vi "Compress.vi"(4 "No of threads":i32, 6 "Compression Level":i32=3, 8 "error in (no error)":errorcluster, 11 "lvzstd in":refnum<class "lvzstd.lvclass">) -> (0 "error out":errorcluster, 3 "lvzstd out":refnum<class "lvzstd.lvclass">)   [LabVIEW 2020, in "lvzstd.lvlib" / "lvzstd.lvclass"]
uses:
  lvzstd.lvclass
  lvzstd.lvclass/lvzstd.ctl
  <vilib>/Utility/error.llb/Error Cluster From Error Code.vi
panel:
  in  "data in":variant
  out "compressed data":string
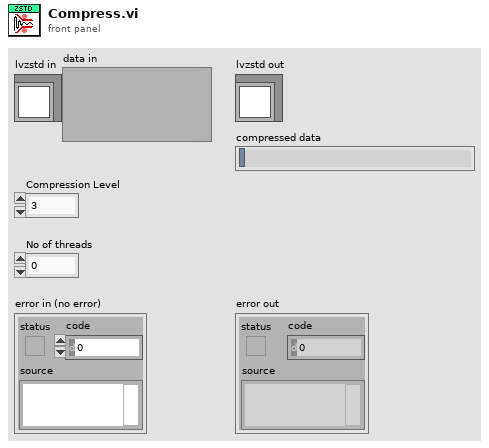
[diagram p1: front panel]
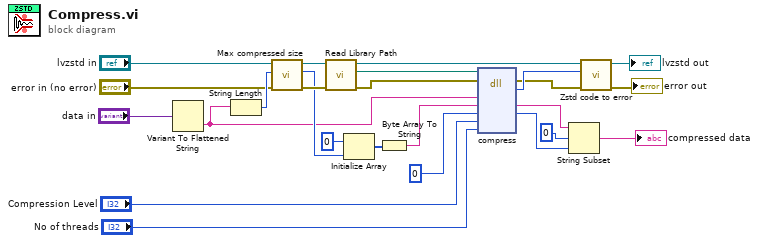
[diagram p0: block diagram]
diagram:
  n1 = Variant To Flattened String(Variant="data in") -> (data string=w2:string)  [unwired: 1 out]
  n2 = String Length(string=w2) -> (length=w25:i32)
  n3 = call-dynamic "Max compressed size.vi"("error in (no error)"="error in (no error)", "source size (bytes)"=w25, "lvzstd in"="lvzstd in") -> ("error out"=w21:errorcluster, "maximum compressed size (bytes)"=w20:i32, "lvzstd out"=w22:refnum<class "lvzstd.lvclass">)  [unwired: 6 in]
  n4 = call "Read Library Path.vi"("error in (no error)"=w21, "lvzstd in"=w22) -> ("error out"=w16:errorcluster, "Library Path"=w17:path, "lvzstd out"=w6:refnum<class "lvzstd.lvclass">)  [unwired: 7 in]
  n5 = Initialize Array(u8 0, w20) -> (w14:u8[])
  n6 = Byte Array To String(unsigned byte array=w14) -> (string=w13:string)
  n7 = dll-call lib="?" fn="compress"(path in=w17, error in=w16, "srcHandle"=w2, "dstHandle"=w13, "compressedSize"=0, "cLevel"="Compression Level", "noThreads"="No of threads") -> (error out=w8:errorcluster, "return type"=w9:i32, "dstHandle"=w4:string, "compressedSize"=w12:i32)  [unwired: 4 in, 1 out]
  n8 = String Subset(string=w4, offset (0)=0, length (rest)=w12) -> (substring=→"compressed data":string)
  n9 = call "Zstd code to error.vi"("error in"=w8, "Error code"=w9, "lvzstd in"=w6) -> ("error in (no error)"=→"error out":errorcluster, "lvzstd out"=→"lvzstd out":refnum<class "lvzstd.lvclass">)  [unwired: 7 in]
